vi "Get Sensor Servo.vi"(8 "error in (no error)":errorcluster, 11 "NI_Robotics_Starter Kit Host in":refnum<class "NI_Robotics_Starter Kit Host.lvclass">) -> (0 "error out":errorcluster, 2 "sensor servo":refnum<class "NI_Robotics_Starter Kit Servo Motor.lvclass">, 3 "NI_Robotics_Starter Kit Host out":refnum<class "NI_Robotics_Starter Kit Host.lvclass">)   [LabVIEW 2017, in "NI_Robotics_Starter Kit Host.lvclass"]
uses:
  <vilib>/robotics/Starter Kit/Host Interface/NI_Robotics_Starter Kit Host.lvclass
  <vilib>/robotics/Starter Kit/Servo Motor/NI_Robotics_Starter Kit Servo Motor.lvclass
  <vilib>/robotics/Starter Kit/Host Interface/NI_Robotics_Starter Kit Host.lvclass/NI_Robotics_Starter Kit Host.ctl
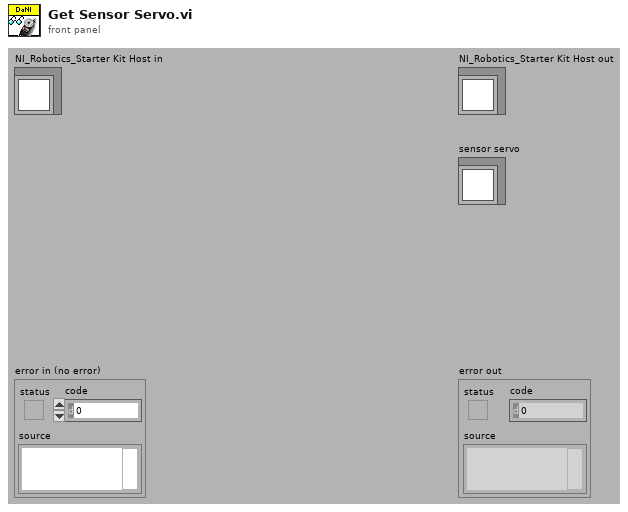
[diagram p1: front panel]
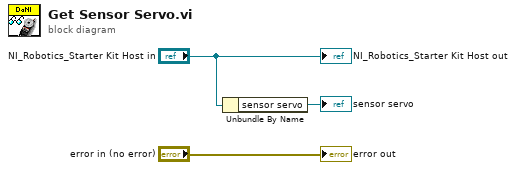
[diagram p0: block diagram]
diagram:
  n1 = Unbundle By Name("NI_Robotics_Starter Kit Host in") -> ("sensor servo"=→"sensor servo":refnum<class "NI_Robotics_Starter Kit Servo Motor.lvclass">)
  "error out" <- "error in (no error)"
  "NI_Robotics_Starter Kit Host out" <- "NI_Robotics_Starter Kit Host in"
